vi "UMLEditor Main.vi"(1 "StartProject":string, 3 "StartTarget":string) -> ()   [LabVIEW 2012] (continued)
            n350 = Index Array(array=w1041) -> (element=w1040:refnum<class "AbstractNode.lvclass">)  [unwired: 1 in]
            n351 = case shown="\"None\", Default" w1043 {
              tunnel: [w1051 w1090 w1128] -> w1044
              tunnel: [w1050 w1086 w1127] -> w1038
              tunnel: w1042 -> [w1049 w1089 w1124]
              tunnel: w1040 -> [_ _ w1126]
              tunnel: w1035 -> [w1048 w1087 w1125]
              tunnel: w1039 -> [w1046 w1085 w1123]
              tunnel: w1037 -> [w1047 _ _]
              tunnel: w1036 -> [w1045 w1088 w1122]
              frame "Edge" {
                n352 = case shown="Default" w1048 {
                  selector: w1048 -> [w1059 _ _]
                  tunnel: w1049 -> [w1061 w1078 w1082]
                  tunnel: w1046 -> [w1054 w1080 w1084]
                  tunnel: [w1056 w1077 w1081] -> w1050
                  tunnel: w1047 -> [w1060 _ _]
                  tunnel: [w1055 w1078 w1082] -> w1051
                  tunnel: w1045 -> [w1052 _ _]
                  frame Default {
                    n353 = call-dynamic "ExecuteMenuCommand.vi"("reference"=w1060, "Command"=w1059, "error in (no error)"=w1061) -> ("reference out"=w1057:refnum<class "AbstractEdge.lvclass">, "EditorAction"=w1058:T45, "error out"=w1053:errorcluster)  [unwired: 14 in]
                    n354 = case shown="\"ExecuteCommand\"" w1058 {
                      tunnel: w1054 -> [w1062 w1067 w1076]
                      tunnel: [w1062 w1066 w1073] -> w1056
                      tunnel: w1057 -> [_ _ _]
                      tunnel: w1053 -> [w1063 w1071 w1074]
                      tunnel: [w1063 w1069 w1074] -> w1055
                      tunnel: w1052 -> [_ w1065 _]
                      frame "NoAction", Default {
                      }
                      frame "Repaint" {
                        n355 = call-dynamic "layout.vi"("reference"=w1065, "error in (no error)"=w1071) -> ("error out"=w1070:errorcluster)  [unwired: 16 in, 1 out]
                        n356 = Bundle By Name(cluster=w1067, "state"=UMLEditor_statesType."Repaint") -> (w1064:T7)
                        n357 = call <resource>:"UMLEditor setDiagramInfo.vi"("error in (no error)"=w1070, "localVariablesIn"=w1064, "action"=enum16{"Name/Dir", "Unsaved", "Saved"}."Unsaved") -> ("localVariablesOut"=w1066:T7, "error out"=w1069:errorcluster)  [unwired: 2 in, 13 out]
                      }
                      frame "ExecuteCommand" {
                        n358 = Bundle By Name(cluster=w1076, "state"=UMLEditor_statesType."ExecuteCommand") -> (w1073:T7)
                      }
                    }
                  }
                  frame "Remove Edge" {
                    n359 = Bundle By Name(cluster=w1080, "state"=UMLEditor_statesType."RemoveSelected") -> (w1077:T7)
                  }
                  frame "Configure Edge" {
                    n360 = Bundle By Name(cluster=w1084, "state"=UMLEditor_statesType."EditSelected") -> (w1081:T7)
                  }
                }
              }
              frame "None", Default {
                n361 = Unbundle By Name(w1085) -> ("graphics"=w1094:refnum<class "Graphics.lvclass">, "grid"=w1093:refnum<class "Grid.lvclass">)
                n362 = Bundle By Name(cluster=w1085, "state"=UMLEditor_statesType."Repaint") -> (w1092:T7)
                n363 = case shown="Default" w1087 {
                  selector: w1087 -> [_ w1107]
                  tunnel: w1089 -> [w1097 w1114]
                  tunnel: [w1097 w1112] -> w1091
                  tunnel: w1094 -> [_ w1106]
                  tunnel: w1093 -> [_ w1105]
                  tunnel: w1092 -> [w1096 w1111]
                  tunnel: [w1096 w1110] -> w1086
                  tunnel: w1088 -> [_ w1108]
                  tunnel: w1085 -> [_ w1098]
                  frame "" {
                  }
                  frame Default {
                    n364 = property on="Picture" class="Pict"() -> ("Mouse"=w1100:T42)  [unwired: 2 in, 2 out]
                    n365 = Unbundle By Name(w1100) -> ("Mouse Position"=w1104:cluster{"X":i32, "Y":i32})
                    n366 = Unbundle By Name(w1098) -> ("zoom"=w1101:dbl, "offset"=w1103:T12)
                    n367 = Add(x=w1103, y=w1104) -> (x+y=w1102:T12)
                    n368 = Divide(x=w1102, y=w1101) -> (x/y=w1099:T12)
                    n369 = call-dynamic "HandleRightClickMenuOption.vi"("reference"=w1108, "MenuOption"=w1107, "graphics"=w1106, "grid"=w1105, "point2D"=w1099, "error in (no error)"=w1114) -> ("Cancel"=w1109:bool, "error out"=w1113:errorcluster)  [unwired: 11 in, 1 out]
                    n370 = case shown="False" w1109 {
                      tunnel: w1113 -> [w1118 w1121]
                      tunnel: [w1117 w1121] -> w1112
                      tunnel: w1111 -> [w1115 w1120]
                      tunnel: [w1116 w1120] -> w1110
                      frame False {
                        n371 = call <resource>:"UMLEditor setDiagramInfo.vi"("error in (no error)"=w1118, "localVariablesIn"=w1115, "action"=enum16{"Name/Dir", "Unsaved", "Saved"}."Unsaved") -> ("localVariablesOut"=w1116:T7, "error out"=w1117:errorcluster)  [unwired: 2 in, 13 out]
                      }
                      frame True {
                      }
                    }
                  }
                }
                n372 = call <resource>:"UMLEditor UpdatesToolbuttons.vi"("error in (no error)"=w1091) -> ("error out"=w1090:errorcluster)  [unwired: 5 in, 13 out]
              }
              frame "Node" {
                n373 = case shown="Default" w1125 {
                  selector: w1125 -> [w1136 _ _]
                  tunnel: w1124 -> [w1138 w1156 w1160]
                  tunnel: w1123 -> [w1131 w1158 w1162]
                  tunnel: [w1133 w1155 w1159] -> w1127
                  tunnel: w1126 -> [w1137 _ _]
                  tunnel: [w1132 w1156 w1160] -> w1128
                  tunnel: w1122 -> [w1129 _ _]
                  frame Default {
                    n374 = call-dynamic "ExecuteMenuCommand.vi"("reference"=w1137, "Command"=w1136, "error in (no error)"=w1138) -> ("EditorAction"=w1135:T45, "FlattenCommandSettings"=w1134:T15, "error out"=w1130:errorcluster)  [unwired: 13 in, 1 out]
                    n375 = case shown="\"ExecuteCommand\"" w1135 {
                      tunnel: w1131 -> [w1139 w1143 w1154]
                      tunnel: [w1139 w1144 w1150] -> w1133
                      tunnel: w1134 -> [_ _ w1152]
                      tunnel: w1130 -> [w1140 w1148 w1151]
                      tunnel: [w1140 w1146 w1151] -> w1132
                      tunnel: w1129 -> [_ w1141 _]
                      frame "NoAction", Default {
                      }
                      frame "Repaint" {
                        n376 = call-dynamic "layout.vi"("reference"=w1141, "error in (no error)"=w1148) -> ("error out"=w1147:errorcluster)  [unwired: 16 in, 1 out]
                        n377 = Bundle By Name(cluster=w1143, "state"=UMLEditor_statesType."Repaint") -> (w1142:T7)
                        n378 = call <resource>:"UMLEditor setDiagramInfo.vi"("error in (no error)"=w1147, "localVariablesIn"=w1142, "action"=enum16{"Name/Dir", "Unsaved", "Saved"}."Unsaved") -> ("localVariablesOut"=w1144:T7, "error out"=w1146:errorcluster)  [unwired: 2 in, 13 out]
                      }
                      frame "ExecuteCommand" {
                        n379 = Bundle By Name(cluster=w1154, "state"=UMLEditor_statesType."ExecuteCommand", "FlattenCommandSettings"=w1152) -> (w1150:T7)
                      }
                    }
                  }
                  frame "Remove Node" {
                    n380 = Bundle By Name(cluster=w1158, "state"=UMLEditor_statesType."RemoveSelected") -> (w1155:T7)
                  }
                  frame "Configure Node" {
                    n381 = Bundle By Name(cluster=w1162, "state"=UMLEditor_statesType."EditSelected") -> (w1159:T7)
                  }
                }
              }
            }
          }
          event "Picture": Shortcut Menu Activation? {
            # "Show right click menus for graphs, node and edges"
            n382 = event-data() -> ("MenuRef"=w1186:refnum<k9>)  [unwired: 1 out]
            n383 = property on="Picture" class="Pict"() -> ("Mouse"=w1180:T42)  [unwired: 2 in, 2 out]
            n384 = Unbundle By Name(w1164) -> ("graphics"=w1168:refnum<class "Graphics.lvclass">)
            n385 = Unbundle By Name(w1180) -> ("Mouse Position"=w1184:cluster{"X":i32, "Y":i32})
            n386 = Delete Menu Items(6:w1185, 9:w1186) -> (0:w1173:errorcluster, 3:w1176:refnum<k9>)  [unwired: 2 out]
            n387 = Unbundle By Name(w1164) -> ("zoom"=w1181:dbl, "offset"=w1183:T12)
            n388 = Add(x=w1183, y=w1184) -> (x+y=w1182:T12)
            n389 = Divide(x=w1182, y=w1181) -> (x/y=w1165:T12)
            n390 = call <resource>:"UMLEditor_FindObject.vi"("offset"=w1165, "error in"=w1173, "graphics"=w1168, "graph"=w1170) -> ("error out"=w1166:errorcluster, "NodeFound"=w1172:bool, "node"=w1171:refnum<class "AbstractNode.lvclass">, "edge"=w1169:refnum<class "AbstractEdge.lvclass">, "EdgeFound"=w1167:bool)  [unwired: 2 in, 1 out]
            n391 = Bundle By Name(cluster=w1164, "lastMousePoint"=w1165) -> (w1163:T7)
            n392 = case shown="False" w1167 {
              tunnel: w1172 -> [w1203 _]
              tunnel: w1171 -> [w1202 _]
              tunnel: [w1201 w1235] -> w1175
              tunnel: w1163 -> [w1200 w1240]
              tunnel: [w1199 w1239] -> w1179
              tunnel: w1170 -> [w1198 _]
              tunnel: w1169 -> [_ w1241]
              tunnel: w1164 -> [w1197 _]
              tunnel: w1165 -> [w1196 _]
              tunnel: [w1195 w1236] -> w1177
              tunnel: w1166 -> [w1194 w1234]
              frame False {
                n393 = case shown="True" w1203 {
                  tunnel: w1202 -> [_ w1227]
                  tunnel: [w1207 w1219] -> w1201
                  tunnel: w1200 -> [w1214 w1225]
                  tunnel: [w1209 w1224] -> w1199
                  tunnel: w1198 -> [w1211 w1223]
                  tunnel: w1197 -> [_ _]
                  tunnel: w1196 -> [_ w1217]
                  tunnel: [w1206 w1220] -> w1195
                  tunnel: w1194 -> [w1204 w1218]
                  frame False {
                    n394 = call-dynamic "GetRightClickMenu.vi"("reference"=w1211, "error in (no error)"=w1204) -> ("Array"=w1206:string[], "error out"=w1208:errorcluster)  [unwired: 14 in, 2 out]
                    n395 = Bundle By Name(cluster=w1214, "selcted"=UMLEditor_tooltype."None", "toolType"=UMLEditor_tooltype."None", "tool"=UMLEditor_toolsType."CD_Select", "state"=UMLEditor_statesType."Repaint", "SelectedNodes"=refnum<class "AbstractNode.lvclass">[] [], "selectedEdge"=refnum<class "AbstractEdge.lvclass"> refnum) -> (w1209:T7)
                    n396 = call <resource>:"UMLEditor UpdatesToolbuttons.vi"("error in (no error)"=w1208) -> ("error out"=w1207:errorcluster)  [unwired: 5 in, 13 out]
                  }
                  frame True {
                    n397 = call-dynamic "GetNodeMenuOptions.vi"("reference"=w1227, "MousePos"=w1217, "error in (no error)"=w1218) -> ("reference out"=w1222:refnum<class "AbstractNode.lvclass">, "MenuOptions"=w1220:string[], "error out"=w1219:errorcluster)  [unwired: 14 in]
                    n398 = Array Size(array=w1220) -> (size(s)=w1226:i32)
                    n399 = Build Array(w1222) -> (w1221:refnum<class "AbstractNode.lvclass">[])
                    n400 = case shown="1.." w1226 {
                      tunnel: w1220 -> [_ _]
                      tunnel: w1225 -> [w1228 w1232]
                      tunnel: [w1228 w1231] -> w1224
                      tunnel: w1221 -> [_ w1230]
                      tunnel: w1223 -> [_ _]
                      frame 0, Default {
                      }
                      frame 1.. {
                        n401 = Bundle By Name(cluster=w1232, "selcted"=UMLEditor_tooltype."Node", "SelectedNodes"=w1230, "state"=UMLEditor_statesType."Repaint") -> (w1231:T7)
                      }
                    }
                  }
                }
              }
              frame True {
                n402 = call-dynamic "GetEdgeMenu.vi"("reference"=w1241, "error in (no error)"=w1234) -> ("reference out"=w1237:refnum<class "AbstractEdge.lvclass">, "MenuOptions"=w1236:string[], "error out"=w1235:errorcluster)  [unwired: 15 in]
                n403 = Array Size(array=w1236) -> (size(s)=w1238:i32)
                n404 = case shown="1.." w1238 {
                  tunnel: w1240 -> [w1242 w1246]
                  tunnel: [w1242 w1244] -> w1239
                  tunnel: w1237 -> [_ w1245]
                  frame 0, Default {
                  }
                  frame 1.. {
                    n405 = Bundle By Name(cluster=w1246, "selcted"=UMLEditor_tooltype."Edge", "selectedEdge"=w1245, "state"=UMLEditor_statesType."Repaint") -> (w1244:T7)
                  }
                }
              }
            }
            n406 = for {
              shift-right: [w1189] -> w1174
              shift-left: w1175 -> [w1191]
              tunnel: w1177 -> [w1190] mode=indexing
              tunnel: w1176 -> [w1187]
              n407 = case shown="Default" w1190 {
                selector: w1190 -> [w1192 _]
                tunnel: [w1192 "APP_SEPARATOR" ("after item")] -> w1188
                frame Default {
                }
                frame "" {
                }
              }
              n408 = Insert Menu Items(6:w1191, 7:w1188, 8:w1188, 9:w1187) -> (0:w1189:errorcluster)  [unwired: 4 out]
            }
            n409 = event-data("Discard?"=FALSE) -> ()  [unwired: 1 in, 1 out]
          }
          event "Picture": Drag Enter {
            n410 = event-data() -> ("Coords"=w1249:T46, "Available Data Names"=w1248:string[])  [unwired: 8 out]
            n411 = stacked-sequence {
              tunnel: w1249 -> [_]
              tunnel: w1248 -> [_]
              frame #0 {
              }
            }
            n412 = event-data("Accepted?"=TRUE) -> ()  [unwired: 1 in, 1 out]
          }
          event Value Change {
            n413 = event-data() -> ("OldVal"=w1255:T1, "NewVal"=w1254:T1)  [unwired: 1 out]
            n414 = Not Equal?(x=w1255, y=w1254) -> (x != y?=w1253:T1)
            n415 = Cluster To Array(cluster=w1253) -> (array=w1280:bool[])
            n416 = Initialize Array(FALSE ("element"), 12 ("dimension size")) -> (w1276:bool[])
            n417 = Search 1D Array(1D array=w1280, element=TRUE) -> (index of element=w1259:i32)  [unwired: 1 out]
            n418 = Replace Array Subset(array=w1276, new element=TRUE ("element"), index=w1259) -> (w1274:bool[])
            n419 = Equal To 0?(x=w1259) -> (x = 0?=w1256:bool)
            n420 = Array To Cluster(array=w1274) -> (cluster=w1273:T47)
            n421 = local write "classDiagramTools"(w1273) -> ()
            n422 = Equal?(x=w1259, y=10) -> (x = y?=w1257:bool)
            n423 = In Range and Coerce(upper limit=3, x=w1259, lower limit=1) -> (In Range?=w1269:bool)  [unwired: 1 out]
            n424 = Or(x=w1269, y=w1257) -> (x .or. y?=w1260:bool)
            n425 = Select(t=UMLEditor_tooltype."Node" ("toolType"), s=w1260, f=UMLEditor_tooltype."Edge" ("toolType")) -> (s? t:f=w1267:T9)
            n426 = Select(t=UMLEditor_tooltype."None" ("toolType"), s=w1256, f=w1267) -> (s? t:f=w1264:T9)
            n427 = case shown="0, Default" w1259 {
              tunnel: [UMLEditor_toolsType."CD_Select" ("tool") UMLEditor_toolsType."CD_Class" ("tool") UMLEditor_toolsType."CD_Interface" ("tool") UMLEditor_toolsType."CD_Package" ("tool") UMLEditor_toolsType."CD_Dependency" ("tool") UMLEditor_toolsType."CD_Inheritance" ("tool") UMLEditor_toolsType."CD_InterfaceImp" ("tool") UMLEditor_toolsType."CD_Association" ("tool") UMLEditor_toolsType."CD_Aggregation" ("tool") UMLEditor_toolsType."CD_Composite" ("tool") UMLEditor_toolsType."CD_Note" ("tool") UMLEditor_toolsType."CD_NoteConn" ("tool")] -> w1261
              frame 0, Default {
              }
              frame 1 {
              }
              frame 2 {
              }
              frame 3 {
              }
              frame 4 {
              }
              frame 5 {
              }
              frame 6 {
              }
              frame 7 {
              }
              frame 8 {
              }
              frame 9 {
              }
              frame 10 {
              }
              frame 11 {
              }
            }
            n428 = Bundle By Name(cluster=w1263, "toolType"=w1264, "tool"=w1261) -> (w1272:T7)
          }
          event Value Change {
            n429 = event-data() -> ("OldVal"=w1295:T3, "NewVal"=w1294:T3)  [unwired: 1 out]
            n430 = Not Equal?(x=w1295, y=w1294) -> (x != y?=w1293:T3)
            n431 = Cluster To Array(cluster=w1293) -> (array=w1311:bool[])
            n432 = Search 1D Array(1D array=w1311, element=TRUE) -> (index of element=w1296:i32)  [unwired: 1 out]
            n433 = Equal To 0?(x=w1296) -> (x = 0?=w1299:bool)
            n434 = Initialize Array(FALSE ("element"), 10 ("dimension size")) -> (w1318:bool[])
            n435 = Equal?(x=w1296, y=8) -> (x = y?=w1300:bool)
            n436 = In Range and Coerce(upper limit=3, x=w1296, lower limit=1) -> (In Range?=w1307:bool)  [unwired: 1 out]
            n437 = Replace Array Subset(array=w1318, new element=TRUE ("element"), index=w1296) -> (w1316:bool[])
            n438 = Or(x=w1307, y=w1300) -> (x .or. y?=w1302:bool)
            n439 = Array To Cluster(array=w1316) -> (cluster=w1315:T48)
            n440 = local write "usecaseDiagramTools"(w1315) -> ()
            n441 = Select(t=UMLEditor_tooltype."Node" ("toolType"), s=w1302, f=UMLEditor_tooltype."Edge" ("toolType")) -> (s? t:f=w1305:T9)
            n442 = Select(t=UMLEditor_tooltype."None" ("toolType"), s=w1299, f=w1305) -> (s? t:f=w1297:T9)
            n443 = case shown="9" w1296 {
              tunnel: [UMLEditor_toolsType."UD_Select" ("tool") UMLEditor_toolsType."UD_System" ("tool") UMLEditor_toolsType."UD_Actor" ("tool") UMLEditor_toolsType."UD_UseCase" ("tool") UMLEditor_toolsType."UD_Assoiciation" ("tool") UMLEditor_toolsType."UD_Generalization" ("tool") UMLEditor_toolsType."UD_GeneralizationIncludes" ("tool") UMLEditor_toolsType."UD_GeneralizationExtends" ("tool") UMLEditor_toolsType."UD_Note" ("tool") UMLEditor_toolsType."UD_NoteEdge" ("tool")] -> w1298
              frame 0, Default {
              }
              frame 1 {
              }
              frame 2 {
              }
              frame 3 {
              }
              frame 4 {
              }
              frame 5 {
              }
              frame 6 {
              }
              frame 7 {
              }
              frame 8 {
              }
              frame 9 {
              }
            }
            n444 = Bundle By Name(cluster=w1313, "toolType"=w1297, "tool"=w1298) -> (w1314:T7)
          }
          event Value Change {
            n445 = event-data() -> ("OldVal"=w1333:T4, "NewVal"=w1332:T4)  [unwired: 1 out]
            n446 = Not Equal?(x=w1333, y=w1332) -> (x != y?=w1331:T4)
            n447 = Cluster To Array(cluster=w1331) -> (array=w1349:bool[])
            n448 = Search 1D Array(1D array=w1349, element=TRUE) -> (index of element=w1335:i32)  [unwired: 1 out]
            n449 = Equal To 0?(x=w1335) -> (x = 0?=w1337:bool)
            n450 = Equal?(x=w1335, y=6) -> (x = y?=w1338:bool)
            n451 = In Range and Coerce(upper limit=4, x=w1335, lower limit=1) -> (In Range?=w1345:bool)  [unwired: 1 out]
            n452 = Initialize Array(FALSE ("element"), 8 ("dimension size")) -> (w1356:bool[])
            n453 = Or(x=w1345, y=w1338) -> (x .or. y?=w1340:bool)
            n454 = Replace Array Subset(array=w1356, new element=TRUE ("element"), index=w1335) -> (w1354:bool[])
            n455 = Array To Cluster(array=w1354) -> (cluster=w1353:T49)
            n456 = Select(t=UMLEditor_tooltype."Node" ("toolType"), s=w1340, f=UMLEditor_tooltype."Edge" ("toolType")) -> (s? t:f=w1343:T9)
            n457 = local write "stateDiagramTools"(w1353) -> ()
            n458 = Select(t=UMLEditor_tooltype."None" ("toolType"), s=w1337, f=w1343) -> (s? t:f=w1336:T9)
            n459 = case shown="4" w1335 {
              tunnel: [UMLEditor_toolsType."STD_Select" ("tool") UMLEditor_toolsType."STD_State" ("tool") UMLEditor_toolsType."STD_InitailState" ("tool") UMLEditor_toolsType."STD_FinalState" ("tool") UMLEditor_toolsType."STD_ChoiseState" ("tool") UMLEditor_toolsType."STD_StateTransation" ("tool") UMLEditor_toolsType."STD_Note" ("tool") UMLEditor_toolsType."STD_NoteEdge" ("tool")] -> w1334
              frame 0, Default {
              }
              frame 1 {
              }
              frame 2 {
              }
              frame 3 {
              }
              frame 4 {
              }
              frame 5 {
              }
              frame 6 {
              }
              frame 7 {
              }
            }
            n460 = Bundle By Name(cluster=w1351, "toolType"=w1336, "tool"=w1334) -> (w1352:T7)
          }
          event Value Change {
            n461 = event-data() -> ("OldVal"=w1369:T2, "NewVal"=w1368:T2)  [unwired: 1 out]
            n462 = Not Equal?(x=w1369, y=w1368) -> (x != y?=w1367:T2)
            n463 = Cluster To Array(cluster=w1367) -> (array=w1385:bool[])
            n464 = Search 1D Array(1D array=w1385, element=TRUE) -> (index of element=w1372:i32)  [unwired: 1 out]
            n465 = Equal To 0?(x=w1372) -> (x = 0?=w1373:bool)
            n466 = Equal?(x=w1372, y=4) -> (x = y?=w1374:bool)
            n467 = In Range and Coerce(upper limit=2, x=w1372, lower limit=1) -> (In Range?=w1381:bool)  [unwired: 1 out]
            n468 = Initialize Array(FALSE ("element"), 6 ("dimension size")) -> (w1392:bool[])
            n469 = Or(x=w1381, y=w1374) -> (x .or. y?=w1376:bool)
            n470 = Replace Array Subset(array=w1392, new element=TRUE ("element"), index=w1372) -> (w1390:bool[])
            n471 = Array To Cluster(array=w1390) -> (cluster=w1389:T50)
            n472 = Select(t=UMLEditor_tooltype."Node" ("toolType"), s=w1376, f=UMLEditor_tooltype."Edge" ("toolType")) -> (s? t:f=w1379:T9)
            n473 = local write "sequenceDiagramTools"(w1389) -> ()
            n474 = Select(t=UMLEditor_tooltype."None" ("toolType"), s=w1373, f=w1379) -> (s? t:f=w1371:T9)
            n475 = case shown="5" w1372 {
              tunnel: [UMLEditor_toolsType."SQD_Select" ("tool") UMLEditor_toolsType."SQD_Object" ("tool") UMLEditor_toolsType."SQD_ActionBar" ("tool") UMLEditor_toolsType."SQD_Call" ("tool") UMLEditor_toolsType."SQD_Note" ("tool") UMLEditor_toolsType."SQD_NoteConn" ("tool")] -> w1370
              frame 0, Default {
              }
              frame 1 {
              }
              frame 2 {
              }
              frame 3 {
              }
              frame 4 {
              }
              frame 5 {
              }
            }
            n476 = Bundle By Name(cluster=w1387, "toolType"=w1371, "tool"=w1370) -> (w1388:T7)
          }
          event "Picture": Mouse Up {
            w1431 = T12 {"x"=nan, "y"=nan} ("rubberBandStart")
            w1404 = FALSE ("b_dwn")
            n477 = event-data() -> ("Mods.Double Click"=w1419:bool, "Coords"=w1413:T46)  [unwired: 1 out]
            n478 = Unbundle By Name(w1412) -> ("CONNECT_THRESHOLD"=w1426:i32)
            n479 = property on="Picture" class="Pict"() -> ("Mouse"=w1416:T42, "Draw Area Size"=w1415:T43, "Origin"=w1414:T44)  [unwired: 2 in, 2 out]
            n480 = Unbundle By Name(w1412) -> ("lastMousePoint"=w1403:T12, "rubberBandStart"=w1427:T12, "selcted"=w1422:T9, "offset"=w1408:T12, "zoom"=w1406:dbl)
            n481 = Unbundle By Name(w1412) -> ("HotSpotCursor"=w1411:bool, "HotSpotFunction"=w1410:T19)
            n482 = Unbundle By Name(w1412) -> ("SelectedNodes"=w1420:refnum<class "AbstractNode.lvclass">[])
            n483 = Unbundle By Name(w1416) -> ("Mouse Position"=w1409:cluster{"X":i32, "Y":i32})
            n484 = call-poly <vilib>:"Set Cursor.vi"("VI reference (current VI)"=w1401, "icon"=u16 1) -> ()  [unwired: 1 in, 9 out]
            n485 = Tick Count (ms)() -> (millisecond timer value=w1418:u32)
            n486 = Add(x=w1409, y=w1408) -> (x+y=w1407:T12)
            n487 = call <resource>:"UMLEditor IsMouseOutsideDrawingArea.vi"("Mouse"=w1416, "Draw Area Size"=w1415, "Origin"=w1414) -> ("OutsideDrawingArea"=w1417:bool)  [unwired: 2 in, 14 out]
            n488 = call <resource>:"Point getValues.vi"("point2D"=w1427) -> ("valid"=w1429:bool)  [unwired: 18 out]
            n489 = Divide(x=w1407, y=w1406) -> (x/y=w1405:T12)
            n490 = case shown="False" w1417 {
              tunnel: w1429 -> [w1450 _]
              tunnel: w1428 -> [w1449 w1712]
              tunnel: w1427 -> [w1448 _]
              tunnel: w1426 -> [w1447 _]
              tunnel: [w1436 w1711] -> w1425
              tunnel: w1424 -> [w1446 _]
              tunnel: [w1445 w1712] -> w1423
              tunnel: w1422 -> [w1444 _]
              tunnel: w1412 -> [w1443 w1711]
              tunnel: UMLEditor_tooltype."None" ("y") -> [w1442 _]
              tunnel: w1420 -> [w1441 _]
              tunnel: w1419 -> [w1440 _]
              tunnel: w1418 -> [w1439 _]
              tunnel: w1413 -> [w1438 _]
              tunnel: w1411 -> [w1437 _]
              tunnel: w1410 -> [w1435 _]
              tunnel: w1405 -> [w1434 _]
              tunnel: w1403 -> [w1433 _]
              frame False {
                n491 = case shown="False" w1437 {
                  tunnel: w1450 -> [w1466 _]
                  tunnel: w1449 -> [w1465 w1666]
                  tunnel: w1448 -> [w1464 _]
                  tunnel: w1447 -> [w1463 _]
                  tunnel: w1446 -> [w1461 w1662]
                  tunnel: [w1460 w1669] -> w1445
                  tunnel: w1444 -> [w1459 _]
                  tunnel: w1443 -> [w1458 w1668]
                  tunnel: w1442 -> [w1457 _]
                  tunnel: w1441 -> [w1456 w1665]
                  tunnel: w1440 -> [w1455 _]
                  tunnel: w1439 -> [w1454 _]
                  tunnel: w1438 -> [w1453 _]
                  tunnel: [w1462 w1667] -> w1436
                  tunnel: w1435 -> [_ w1664]
                  tunnel: w1434 -> [w1452 w1663]
                  tunnel: w1433 -> [w1451 _]
                  frame False {
                    n492 = case shown="False" w1466 {
                      tunnel: w1465 -> [w1479 w1574]
                      tunnel: w1458 -> [w1480 w1573]
                      tunnel: w1464 -> [_ w1569]
                      tunnel: w1463 -> [_ w1572]
                      tunnel: w1458 -> [w1476 w1567]
                      tunnel: [w1475 w1571] -> w1462
                      tunnel: w1461 -> [w1477 w1570]
                      tunnel: [w1478 w1568] -> w1460
                      tunnel: w1459 -> [w1474 w1566]
                      tunnel: w1457 -> [w1471 _]
                      tunnel: w1456 -> [w1470 _]
                      tunnel: w1455 -> [w1469 _]
                      tunnel: w1454 -> [_ _]
                      tunnel: w1453 -> [_ w1565]
                      tunnel: w1452 -> [w1468 w1564]
                      tunnel: w1451 -> [w1467 _]
                      frame False {
                        # "Try to lock Assoc to grid is offset is used"
                        n493 = Not Equal?(x=w1474, y=w1471) -> (x != y?=w1473:bool)
                        n494 = And(x=w1473, y=w1469) -> (x .and. y?=w1472:bool)
                        n495 = case shown="False" w1472 {
                          tunnel: w1474 -> [w1491 w1553]
                          tunnel: w1480 -> [w1490 _]
                          tunnel: w1479 -> [w1489 w1555]
                          tunnel: [w1488 w1555] -> w1478
                          tunnel: w1477 -> [w1487 _]
                          tunnel: w1476 -> [w1486 w1557]
                          tunnel: [w1485 w1556] -> w1475
                          tunnel: w1470 -> [w1484 w1554]
                          tunnel: w1468 -> [w1483 _]
                          tunnel: w1468 -> [w1482 _]
                          tunnel: w1467 -> [w1481 _]
                          frame False {
                            n496 = case shown="\"Node\"" w1491 {
                              tunnel: w1490 -> [_ w1504 _]
                              tunnel: w1489 -> [w1493 w1503 w1511]
                              tunnel: [w1493 w1501 w1512] -> w1488
                              tunnel: w1487 -> [_ w1500 w1509]
                              tunnel: w1486 -> [w1492 w1496 w1514]
                              tunnel: [w1492 w1495 w1513] -> w1485
                              tunnel: w1484 -> [_ _ w1508]
                              tunnel: w1483 -> [_ _ w1510]
                              tunnel: w1482 -> [_ _ w1507]
                              tunnel: w1481 -> [_ _ w1506]
                              frame Default {
                              }
                              frame "Edge" {
                                n497 = Unbundle By Name(w1504) -> ("selectedEdge"=w1502:refnum<class "AbstractEdge.lvclass">, "graphics"=w1499:refnum<class "Graphics.lvclass">, "grid"=w1498:refnum<class "Grid.lvclass">)
                                n498 = Bundle By Name(cluster=w1496, "SelectedNodes"=refnum<class "AbstractNode.lvclass">[] [], "state"=UMLEditor_statesType."Repaint") -> (w1495:T7)
                                n499 = call-dynamic "Layout.vi"("reference"=w1502, "graph"=w1500, "graphics"=w1499, "grid"=w1498, "error in (no error)"=w1503) -> ("error out"=w1501:errorcluster)  [unwired: 13 in, 1 out]
                              }
                              frame "Node" {
                                n500 = case shown="True" TRUE {
                                tunnel: [w1516 w1527] -> w1512
                                tunnel: w1511 -> [w1516 w1526]
                                tunnel: w1510 -> [_ w1525]
                                tunnel: w1509 -> [_ w1523]
                                tunnel: w1508 -> [_ w1517]
                                frame False {
                                }
                                frame True {
                                n501 = for {
                                tunnel: w1525 -> [w1538]
                                tunnel: w1523 -> [w1536]
                                shift-right: [w1537] -> w1524
                                shift-left: w1526 -> [w1539]
                                tunnel: w1517 -> [w1535] mode=indexing
                                shift-right: [w1533] -> w1521
                                shift-left: FALSE -> [w1534]
                                shift-right: [w1529] -> w1519
                                shift-left: refnum<class "AbstractNode.lvclass"> refnum ("container") -> [w1530]
                                tunnel: w1517 -> [w1528]
                                n502 = call-dynamic "contains.vi"("reference"=w1536, "node"=w1535, "point2D"=w1538, "error in (no error)"=w1539, "IgnoreNodes"=w1528) -> ("contains"=w1532:bool, "container"=w1531:refnum<class "AbstractNode.lvclass">, "error out"=w1537:errorcluster)  [unwired: 11 in, 1 out]
                                n503 = Or(x=w1534, y=w1532) -> (x .or. y?=w1533:bool)
                                n504 = Select(t=w1531, s=w1532, f=w1530) -> (s? t:f=w1529:refnum<class "AbstractNode.lvclass">)
                                }
                                n505 = case shown="True" w1521 {
                                tunnel: [w1540 w1541] -> w1522
                                tunnel: w1517 -> [_ w1546]
                                tunnel: w1524 -> [w1540 w1545]
                                tunnel: w1519 -> [_ w1544]
                                tunnel: w1523 -> [_ w1542]
                                frame False {
                                }
                                frame True {
                                n506 = for {
                                tunnel: w1546 -> [w1551] mode=indexing
                                shift-right: [w1550] -> w1543
                                shift-left: w1545 -> [w1549]
                                tunnel: [w1548] -> _
                                tunnel: w1544 -> [w1547]
                                n507 = call-dynamic "addNode.vi"("reference"=w1547, "node"=w1551, "error in (no error)"=w1549) -> ("added"=w1548:bool, "error out"=w1550:errorcluster)  [unwired: 14 in, 1 out]
                                }
                                n508 = call-dynamic "RearrangeNodes.vi"("reference in"=w1542, "error in (no error)"=w1543) -> ("error out"=w1541:errorcluster)  [unwired: 16 in, 1 out]
                                }
                                }
                                n509 = call-dynamic "layout.vi"("reference"=w1523, "LayoutNodes(Empty=All)"=w1517, "error in (no error)"=w1522) -> ("error out"=w1527:errorcluster)  [unwired: 15 in, 1 out]
                                }
                                }
                                n510 = Not Equal?(x=w1506, y=w1507) -> ()  [unwired: 1 out]
                                n511 = Bundle By Name(cluster=w1514, "state"=UMLEditor_statesType."Repaint") -> (w1513:T7)
                              }
                            }
                          }
                          frame True {
                            n512 = case shown="True" FALSE {
                              tunnel: w1557 -> [w1558 w1562]
                              tunnel: [w1558 w1561] -> w1556
                              tunnel: w1554 -> [_ w1560]
                              tunnel: w1553 -> [_ w1559]
                              frame False {
                              }
                              frame True {
                                (unwired) UMLEditor_tooltype."Node" ("selcted")
                                n513 = Bundle By Name(cluster=w1562, "selcted"=w1559, "SelectedNodes"=w1560, "state"=UMLEditor_statesType."EditSelected") -> (w1561:T7)
                              }
                            }
                          }
                        }
                      }
                      frame True {
                        n514 = case shown="\"None\", \"Node\"" w1566 {
                          tunnel: w1574 -> [w1599 w1621]
                          tunnel: w1573 -> [_ w1620]
                          tunnel: w1572 -> [_ w1615]
                          tunnel: [w1596 w1614] -> w1571
                          tunnel: w1570 -> [w1598 w1603]
                          tunnel: w1569 -> [w1577 w1612]
                          tunnel: [w1590 w1609] -> w1568
                          tunnel: w1567 -> [w1597 w1606]
                          tunnel: w1565 -> [_ w1601]
                          tunnel: w1564 -> [w1575 w1600]
                          frame "None", "Node" {
                            n515 = Unbundle(w1577) -> ("x"=w1585:dbl, "y"=w1581:dbl)
                            n516 = Unbundle(w1575) -> ("x"=w1584:dbl, "y"=w1580:dbl)
                            n517 = Max & Min(x=w1585, y=w1584) -> (max(x,y)=w1583:dbl, min(x,y)=w1582:dbl)
                            n518 = Max & Min(x=w1581, y=w1580) -> (max(x,y)=w1579:dbl, min(x,y)=w1578:dbl)
                            n519 = Subtract(x=w1583, y=w1582) -> (x-y=w1587:dbl)
                            n520 = Subtract(x=w1579, y=w1578) -> (x-y=w1586:dbl)
                            n521 = Bundle By Name(cluster=T13 {"x"=0.0, "y"=0.0, "width"=0.0, "height"=0.0} ("rectangle"), "x"=w1582, "y"=w1578, "width"=w1587, "height"=w1586) -> (w1576:T13)
                            n522 = call-dynamic "findNodes.vi"("reference"=w1598, "bounds"=w1576, "error in (no error)"=w1599) -> ("Nodes"=w1591:refnum<class "AbstractNode.lvclass">[], "AnyFound"=w1595:bool, "error out"=w1590:errorcluster)  [unwired: 12 in, 2 out]
                            n523 = Select(t=UMLEditor_tooltype."Node" ("selcted"), s=w1595, f=UMLEditor_tooltype."None" ("selcted")) -> (s? t:f=w1594:T9)
                            n524 = Bundle By Name(cluster=w1597, "SelectedNodes"=w1591, "selcted"=w1594, "state"=UMLEditor_statesType."Repaint") -> (w1596:T7)
                          }
                          frame Default {
                            n525 = call <resource>:"UMLEditor ToolBarSettings.vi"("localVariables"=w1620, "error in (no error)"=w1621) -> ("tools"=w1602:T10, "prototypeEdge"=w1619:refnum<class "AbstractEdge.lvclass">, "error out"=w1618:errorcluster)  [unwired: 2 in, 13 out]
                            n526 = call-dynamic "clone.vi"("reference"=w1619, "error in (no error)"=w1618) -> ("clonedEdge"=w1610:refnum<class "AbstractEdge.lvclass">, "error out"=w1617:errorcluster)  [unwired: 15 in, 1 out]
                            n527 = call <resource>:"Point getDistance.vi"("point1"=w1612, "point2"=w1600, "error in (no error)"=w1617) -> ("distance"=w1616:dbl, "error out"=w1613:errorcluster)  [unwired: 15 out]
                            n528 = Greater?(x=w1616, y=w1615) -> (0:w1607:bool)
                            n529 = case shown="True" w1607 {
                              tunnel: w1613 -> [w1622 w1630]
                              tunnel: w1603 -> [_ w1629]
                              tunnel: w1612 -> [_ w1628]
                              tunnel: w1600 -> [_ w1627]
                              tunnel: [w1622 w1626] -> w1611
                              tunnel: w1610 -> [_ w1625]
                              tunnel: [FALSE ("connected") w1624] -> w1608
                              frame False {
                              }
                              frame True {
                                n530 = call-dynamic "connect.vi"("reference"=w1629, "egde"=w1625, "p1"=w1628, "p2"=w1627, "error in (no error)"=w1630) -> ("connected"=w1624:bool, "error out"=w1626:errorcluster)  [unwired: 12 in, 1 out]
                              }
                            }
                            n531 = Bundle By Name(cluster=w1606, "state"=UMLEditor_statesType."Repaint") -> (w1604:T7)
                            n532 = case shown="False" w1608 {
                              tunnel: [w1632 w1645] -> w1614
                              tunnel: w1611 -> [w1636 w1640]
                              tunnel: w1610 -> [w1635 w1642]
                              tunnel: [w1634 w1644] -> w1609
                              tunnel: w1604 -> [w1633 w1643]
                              tunnel: w1603 -> [_ w1641]
                              tunnel: w1602 -> [_ w1638]
                              tunnel: w1601 -> [_ w1637]
                              frame False {
                                n533 = call-dynamic "Destroy.vi"("reference"=w1635, "error in (no error)"=w1636) -> ("error out"=w1634:errorcluster)  [unwired: 16 in, 1 out]
                                n534 = Bundle By Name(cluster=w1633, "selcted"=UMLEditor_tooltype."None") -> (w1632:T7)
                              }
                              frame True {
                                n535 = case shown="\"CD_Aggregation\", \"CD_Composite\"" w1638 {
                                tunnel: w1642 -> [w1653 w1661]
                                tunnel: w1641 -> [w1654 w1660]
                                tunnel: w1640 -> [w1655 w1659]
                                tunnel: [w1652 w1658] -> w1639
                                tunnel: w1637 -> [w1650 _]
                                frame "CD_Aggregation", "CD_Composite" {
                                n536 = call <resource>:"UMLEditor ShowAggregationDialog.vi"("graph"=w1654, "ClassAggregation"=w1653, "error in (no error)"=w1655) -> ("Show"=w1651:bool, "error out"=w1652:errorcluster)  [unwired: 15 out]
                                n537 = case shown="True" w1651 {
                                tunnel: w1650 -> [_ w1657]
                                frame False {
                                }
                                frame True {
                                n538 = call <resource>:"UMLEditor_AggregationClusterDialogControl.vi"("Position"=w1657, "Action(SelectSelect)"=T22."CreateAggregation") -> ()  [unwired: 7 in, 11 out]
                                }
                                }
                                }
                                frame Default {
                                n539 = call <resource>:"UMLEditor CreateNoteText.vi"("graph"=w1660, "NoteEdge?"=w1661, "error in (no error)"=w1659) -> ("error out"=w1658:errorcluster)  [unwired: 16 out]
                                }
                                }
                                n540 = Bundle By Name(cluster=w1643, "modified"=TRUE, "selcted"=UMLEditor_tooltype."Edge", "selectedEdge"=w1642) -> (w1646:T7)
                                n541 = call <resource>:"UMLEditor setDiagramInfo.vi"("error in (no error)"=w1639, "localVariablesIn"=w1646, "action"=enum16{"Name/Dir", "Unsaved", "Saved"}."Unsaved") -> ("localVariablesOut"=w1645:T7, "error out"=w1644:errorcluster)  [unwired: 2 in, 13 out]
                              }
                            }
                          }
                        }
                      }
                    }
                  }
                  frame True {
                    n542 = Bundle By Name(cluster=w1668, "HotSpotCursor"=FALSE) -> (w1670:T7)
                    n543 = case shown="Default" w1664 {
                      tunnel: w1670 -> [w1674 w1689]
                      tunnel: [w1678 w1688] -> w1669
                      tunnel: [w1673 w1687] -> w1667
                      tunnel: w1666 -> [w1680 w1686]
                      tunnel: w1664 -> [_ w1685]
                      tunnel: w1665 -> [w1677 w1684]
                      tunnel: w1663 -> [w1672 w1682]
                      tunnel: w1662 -> [w1679 w1681]
                      frame Default {
                        n544 = call-dynamic "layout.vi"("reference"=w1679, "LayoutNodes(Empty=All)"=w1677, "error in (no error)"=w1680) -> ("error out"=w1678:errorcluster)  [unwired: 15 in, 1 out]
                        n545 = Bundle By Name(cluster=w1674, "newSelected"=FALSE ("HotSpotCursor"), "state"=UMLEditor_statesType."Repaint", "lastMousePoint"=w1672) -> (w1673:T7)
                      }
                      frame "Expand", "Collaps" {
                        n546 = Array Size(array=w1684) -> (size(s)=w1683:i32)
                        n547 = case shown="0, Default" w1683 {
                          tunnel: w1689 -> [w1690 w1699]
                          tunnel: [w1691 w1696] -> w1688
                          tunnel: [w1690 w1705] -> w1687
                          tunnel: w1686 -> [w1691 w1704]
                          tunnel: w1685 -> [_ w1703]
                          tunnel: w1684 -> [_ w1702]
                          tunnel: w1682 -> [_ w1698]
                          tunnel: w1681 -> [_ w1695]
                          frame 0, Default {
                          }
                          frame 1.. {
                            n548 = Index Array(array=w1702) -> (element=w1708:refnum<class "AbstractNode.lvclass">)  [unwired: 1 in]
                            n549 = Equal?(x=w1703, y=UMLEditor_HotSpotType."Collaps") -> (x = y?=w1709:bool)
                            n550 = call-dynamic "Collaps.vi"("reference in"=w1708, "Collaps"=w1709, "error in (no error)"=w1704) -> ("reference out"=w1694:refnum<class "AbstractNode.lvclass">, "error out"=w1707:errorcluster)  [unwired: 15 in]
                            n551 = Bundle By Name(cluster=w1699, "newSelected"=FALSE ("HotSpotCursor"), "state"=UMLEditor_statesType."Repaint", "lastMousePoint"=w1698) -> (w1700:T7)
                            n552 = Build Array(w1694) -> (w1693:refnum<class "AbstractNode.lvclass">[])
                            n553 = call <resource>:"UMLEditor setDiagramInfo.vi"("error in (no error)"=w1707, "localVariablesIn"=w1700, "action"=enum16{"Name/Dir", "Unsaved", "Saved"}."Unsaved") -> ("localVariablesOut"=w1705:T7, "error out"=w1697:errorcluster)  [unwired: 2 in, 13 out]
                            n554 = call-dynamic "layout.vi"("reference"=w1695, "LayoutNodes(Empty=All)"=w1693, "error in (no error)"=w1697) -> ("error out"=w1696:errorcluster)  [unwired: 15 in, 1 out]
                          }
                        }
                      }
                    }
                  }
                }
              }
              frame True {
              }
            }
            n555 = Bundle By Name(cluster=w1425, "ShiftDown"=w1404, "CtrlDown"=w1404, "butDwn"=w1404, "rubberBandStart"=w1431, "dragStartPoint"=w1431, "dragStartBounds"=T13 {"x"=nan, "y"=nan, "width"=nan, "height"=nan}) -> (w1432:T7)
          }
          event Timeout {
            # "MouseDrag"
            n556 = event-data() -> ()  [unwired: 2 out]
            n557 = case shown="True" w1719 {
              tunnel: [w1730 w2066] -> w1714
              tunnel: w1718 -> [w1724 w2039]
              tunnel: w1717 -> [w1732 w2059]
              tunnel: [w1733 w2060] -> w1716
              tunnel: w1715 -> [w1731 w2045]
              tunnel: w1713 -> [w1720 _]
              frame False {
                n558 = property on="Picture" class="Pict"() -> ("Mouse"=w1728:T42)  [unwired: 2 in, 2 out]
                n559 = Unbundle By Name(w1728) -> ("Mouse Position"=w1723:cluster{"X":i32, "Y":i32}, "Mouse Modifiers.Shift Mod"=w1729:bool, "Mouse Modifiers.Menu Mod"=w1727:bool)
                n560 = Unbundle By Name(w1724) -> ("zoom"=w1721:dbl, "offset"=w1726:T12)
                n561 = Add(x=w1726, y=w1723) -> (x+y=w1725:T12)
                n562 = Divide(x=w1725, y=w1721) -> (x/y=w1722:T12)
                n563 = case shown="False" w1729 {
                  tunnel: w1732 -> [w1741 w2013]
                  tunnel: [w1740 w2024] -> w1733
                  tunnel: w1724 -> [w1738 w2014]
                  tunnel: w1731 -> [w1737 w2012]
                  tunnel: [w1742 w2014] -> w1730
                  tunnel: w1727 -> [w1739 _]
                  tunnel: w1722 -> [w1736 _]
                  tunnel: w1721 -> [w1735 _]
                  tunnel: w1720 -> [w1734 _]
                  frame False {
                    n564 = Unbundle By Name(w1738) -> ("ResizePanelInProgress"=w1743:bool)
                    n565 = case shown="False" w1743 {
                      tunnel: w1738 -> [w1765 w1999]
                      tunnel: [w1755 w1997] -> w1742
                      tunnel: w1741 -> [w1769 w1995]
                      tunnel: [w1772 w1995] -> w1740
                      tunnel: w1738 -> [w1776 _]
                      tunnel: w1739 -> [w1773 _]
                      tunnel: w1738 -> [w1767 _]
                      tunnel: w1737 -> [w1770 _]
                      tunnel: w1736 -> [w1759 _]
                      tunnel: w1735 -> [w1752 _]
                      tunnel: w1734 -> [w1744 _]
                      frame False {
                        # "Could generate Error when hibernating"
                        n566 = call <resource>:"GOOP_MouseFunctions.vi"("error in (no error)"=w1769) -> ("button info"=w1751:T51, "axis info"=w1768:T52)  [unwired: 8 in, 1 out]
                        n567 = Unbundle By Name(w1767) -> ("ObjectHotspots"=w1758:T18[])
                        n568 = Unbundle By Name(w1776) -> ("NodesBounds"=w1775:T13)
                        n569 = Unbundle By Name(w1767) -> ("KeyPressTime"=w1764:u32)
                        n570 = Unbundle By Name(w1775) -> ("height"=w1774:dbl, "width"=w1771:dbl)
                        n571 = Unbundle By Name(w1768) -> ("Scrolling"=w1749:i32)
                        n572 = Tick Count (ms)() -> (millisecond timer value=w1766:u32)
                        n573 = Equal To 0?(x=w1764) -> (x = 0?=w1763:bool)
                        n574 = Subtract(x=w1766, y=w1764) -> (x-y=w1762:u32)
                        n575 = feedback-in #1(w1749) -> ()
                        n576 = feedback #1(w1749) -> (w1750:i32)
                        n577 = Select(t=u32 0, s=w1763, f=w1762) -> (s? t:f=w1761:u32)
                        n578 = Subtract(x=w1749, y=w1750) -> (x-y=w1745:i32)
                        n579 = Not Equal To 0?(x=w1749) -> (x != 0?=w1748:bool)
                        n580 = Not Equal To 0?(x=w1745) -> (x != 0?=w1747:bool)
                        n581 = And(x=w1748, y=w1747) -> (x .and. y?=w1746:bool)
                        n582 = case shown="0..750" w1761 {
                          tunnel: w1765 -> [w1781 w1782]
                          tunnel: [w1777 w1782] -> w1757
                          frame Default {
                            n583 = property on="SearchString" class="Str"("Visible"=FALSE) -> ()  [unwired: 2 in, 2 out]
                            n584 = local write "SearchString"("" ("SearchString")) -> ()
                            n585 = Bundle By Name(cluster=w1781, "KeyPressTime"=u32 0) -> (w1777:T7)
                          }
                          frame 0..750 {
                          }
                        }
                        n586 = case shown="False" w1746 {
                          tunnel: w1774 -> [_ w1934]
                          tunnel: w1773 -> [_ w1933]
                          tunnel: w1757 -> [w1795 w1932]
                          tunnel: [w1794 w1931] -> w1756
                          tunnel: [w1789 w1930] -> w1772
                          tunnel: w1769 -> [w1790 w1929]
                          tunnel: w1771 -> [_ w1928]
                          tunnel: w1767 -> [w1788 w1927]
                          tunnel: w1768 -> [w1797 _]
                          tunnel: w1751 -> [w1796 _]
                          tunnel: w1770 -> [w1793 _]
                          tunnel: w1759 -> [w1792 _]
                          tunnel: w1758 -> [w1791 _]
                          tunnel: [w1787 _] -> w1754
                          tunnel: [w1786 _] -> w1753
                          tunnel: w1752 -> [w1784 _]
                          tunnel: w1745 -> [_ w1925]
                          tunnel: w1744 -> [w1783 _]
                          frame False {
                            n587 = call <resource>:"UMLEditor_OnHotSpot.vi"("ZoomLevel"=w1784, "ObjectHotspots"=w1791, "Mouse Position"=w1792) -> ("Function"=w1786:T19, "HotSpotCursor"=w1787:bool, "Node"=w1785:refnum<class "AbstractNode.lvclass">)  [unwired: 5 in, 1 out]
                            n588 = case shown="False" w1787 {
                              tunnel: w1797 -> [w1818 _]
                              tunnel: w1796 -> [w1815 _]
                              tunnel: w1795 -> [w1814 w1907]
                              tunnel: [w1813 w1906] -> w1794
                              tunnel: w1793 -> [w1806 _]
                              tunnel: w1790 -> [w1800 w1910]
                              tunnel: [w1800 w1909] -> w1789
                              tunnel: w1788 -> [_ w1908]
                              tunnel: w1786 -> [_ w1905]
                              tunnel: w1785 -> [_ w1904]
                              tunnel: w1783 -> [w1801 w1903]
                              frame False {
                                n589 = Unbundle By Name(w1818) -> ("Horizontal"=w1817:i32, "Vertical"=w1816:i32)
                                n590 = property on="Project" class="Ring (strict)"() -> ("Strings []"=w1807:string[])  [unwired: 2 in, 2 out]
                                n591 = Unbundle By Name(w1815) -> ("button 1"=w1803:bool)
                                n592 = local read "Project"() -> (w1798:u16)
                                n593 = Index Array(array=w1807, index=w1798) -> (element=w1799:string)
                                n594 = Match Pattern(string=w1799, regular expression="^Untitled") -> (offset past match=w1810:i32)  [unwired: 4 out]
                                n595 = case shown="False" w1803 {
                                tunnel: [_ w1821] -> w1804
                                frame False {
                                }
                                frame True {
                                n596 = call <resource>:"UMLEditor_GetActiveWindow.vi"() -> ("Project Explorer"=w1821:bool)  [unwired: 1 in, 10 out]
                                }
                                }
                                n597 = case shown="False" FALSE {
                                tunnel: w1817 -> [w1826 w1848]
                                tunnel: w1816 -> [w1825 w1847]
                                tunnel: w1804 -> [w1824 w1846]
                                tunnel: [w1823 w1845] -> w1812
                                tunnel: w1803 -> [w1822 w1844]
                                frame True {
                                n598 = while {
                                shift-right: [w1832] -> _
                                shift-left: _ -> [w1831]
                                tunnel: w1826 -> [w1835]
                                tunnel: w1825 -> [w1834]
                                tunnel: w1824 -> [w1832]
                                tunnel: [w1833] -> w1823
                                tunnel: w1822 -> [w1829]
                                stop <- TRUE stop-if-true
                                # "Mouse inside VI"
                                n599 = property class="VI"() -> ("Front Panel.WinBounds"=w1843:T53, "Front Panel.IsFrontmost"=w1827:bool)  [unwired: 2 in, 2 out]
                                n600 = Not(x=w1827) -> (.not. x?=w1828:bool)
                                n601 = Unbundle(w1843) -> ("Left"=w1842:i16, "Top"=w1839:i16, "Right"=w1841:i16, "Bottom"=w1840:i16)
                                n602 = property on="DragAndDropPath" class="Path"("Visible"=w1828) -> ()  [unwired: 2 in, 2 out]
                                n603 = In Range and Coerce(upper limit=w1841, x=w1835, lower limit=w1842) -> (In Range?=w1838:bool)  [unwired: 1 out]
                                n604 = In Range and Coerce(upper limit=w1840, x=w1834, lower limit=w1839) -> (In Range?=w1837:bool)  [unwired: 1 out]
                                n605 = And(x=w1838, y=w1837) -> (x .and. y?=w1830:bool)
                                n606 = Compound Arithmetic op=AND(w1830, invert w1829, w1831) -> (w1833:bool)
                                }
                                }
                                frame False {
                                n607 = while {
                                shift-right: [w1852] -> _
                                shift-left: _ -> [w1851]
                                tunnel: w1848 -> [w1855]
                                tunnel: w1847 -> [w1854]
                                tunnel: w1846 -> [w1852]
                                tunnel: [w1853] -> w1845
                                tunnel: w1844 -> [w1849]
                                stop <- TRUE stop-if-true
                                # "Mouse inside VI"
                                n608 = property class="VI" props=["Front Panel.WinBounds", "Front Panel.IsFrontmost"]() -> ("Front Panel.WinBounds"=w1863:T53)  [unwired: 2 in, 3 out]
                                n609 = Unbundle(w1863) -> ("Left"=w1862:i16, "Top"=w1859:i16, "Right"=w1861:i16, "Bottom"=w1860:i16)
                                n610 = In Range and Coerce(upper limit=w1861, x=w1855, lower limit=w1862) -> (In Range?=w1858:bool)  [unwired: 1 out]
                                n611 = In Range and Coerce(upper limit=w1860, x=w1854, lower limit=w1859) -> (In Range?=w1857:bool)  [unwired: 1 out]
                                n612 = And(x=w1858, y=w1857) -> (x .and. y?=w1850:bool)
                                n613 = Compound Arithmetic op=AND(w1850, invert w1849, w1851) -> (w1853:bool)
                                }
                                }
                                }
                                n614 = while {
                                shift-right: [w1899] -> w1820
                                shift-left: _ -> [w1901]
                                stop <- TRUE stop-if-true
                                n615 = Increment(x=w1901) -> (x+1=w1900:u8)
                                n616 = To Unsigned Byte Integer(number=w1900) -> (unsigned 8bit integer=w1899:u8)
                                }
                                n617 = Empty String/Path?(string/path=w1799) -> (empty?=w1819:bool)
                                n618 = Greater Or Equal To 0?(x=w1810) -> (x >= 0?=w1809:bool)
                                n619 = call-poly <vilib>:"Set Cursor.vi"("error in (no error)"=w1800, "VI reference (current VI)"=w1801, "icon"=u16 1) -> ()  [unwired: 9 out]
                                n620 = Or(x=w1819, y=w1809) -> (x .or. y?=w1808:bool)
                                n621 = case shown="0" w1820 {
